vi "Formula(Scalar).vi"(6 "式":T1, 8 "error in (no error)":errorcluster caption="エラー入力（エラーなし）", 9 "B(値)":dbl, 10 "A(列位置 0～)":u16, 11 "元データ(2D)":string[][](array[string])) -> (0 "error out":errorcluster caption="エラー出力", 3 "結果データ(1D)":dbl[](array[numeric]))   [LabVIEW 2014]
uses:
  EnumFormula.ctl
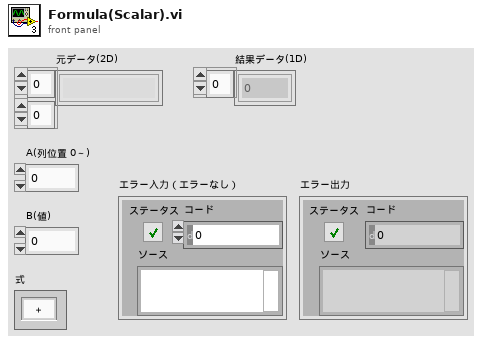
[diagram p1: front panel]
types:
  T1 = typedef "EnumFormula.ctl" = enum16{"＋", "－", "×"}
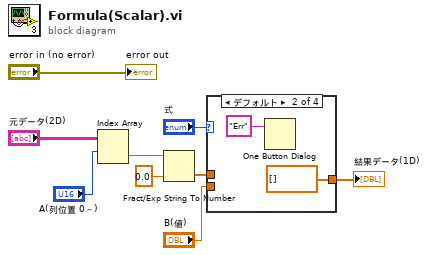
[diagram p0: block diagram]
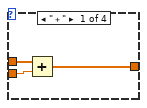
[diagram p2: hidden frame]
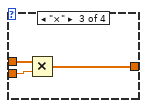
[diagram p3: hidden frame]
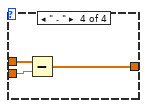
[diagram p4: hidden frame]
diagram:
  n1 = Index Array(array="元データ(2D)", index (row)="A(列位置 0～)") -> (element=w4:string[])  [unwired: 1 in]
  n2 = Fract/Exp String To Number(string=w4, default (0 dbl)=0.0 ("デフォルト（0 I32）")) -> (number=w6:dbl[])  [unwired: 2 in, 1 out]
  n3 = case shown="デフォルト" "式" {
    tunnel: "B(値)" -> [w11 _ w16 w19]
    tunnel: w6 -> [w12 _ w17 w20]
    tunnel: [w10 dbl[] [] w15 w18] -> w7
    frame "＋" {
      # "足し算"
      n4 = Add(x=w12, y=w11) -> (x+y=w10:dbl[])
    }
    frame Default {
      n5 = One Button Dialog(message="Err" ("メッセージ")) -> ()  [unwired: 1 in, 1 out]
    }
    frame "×" {
      n6 = Multiply(x=w17, y=w16) -> (x*y=w15:dbl[])
    }
    frame "－" {
      # "引き算"
      n7 = Subtract(x=w20, y=w19) -> (x-y=w18:dbl[])
    }
  }
  "結果データ(1D)" <- w7
  "error out" <- "error in (no error)"
